vi "Configure USB Address.vi"(5 "Retry Attempts (0)":i32 min=0, 7 "Current Address (-1)":i32=-1, 8 "error in (no error)":errorcluster, 10 "New Address":i32, 11 "VISA resource name (in)":refnum<visa-resource-name>) -> (0 "error out":errorcluster, 2 "Response Cluster":T1 {"Command ID" format="%x"}, 3 "VISA resource name (out)":refnum<visa-resource-name>)   [LabVIEW 2020, in "Omega Platinum Series.lvlib"]
doc: "Change the serial address of a controller. Must be in the range 0-199 (decimal)"
uses:
  Omega Platinum Series.lvlib
  Type Defs/Response.ctl
panel:
  out "Command":string
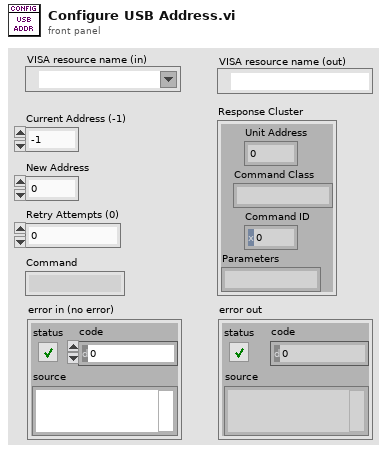
[diagram p1: front panel]
types:
  T1 = typedef "Omega Platinum Series.lvlib/Response.ctl" = cluster{"Unit Address":i32, "Command Class":string, "Command ID":u32, "Parameters":string}
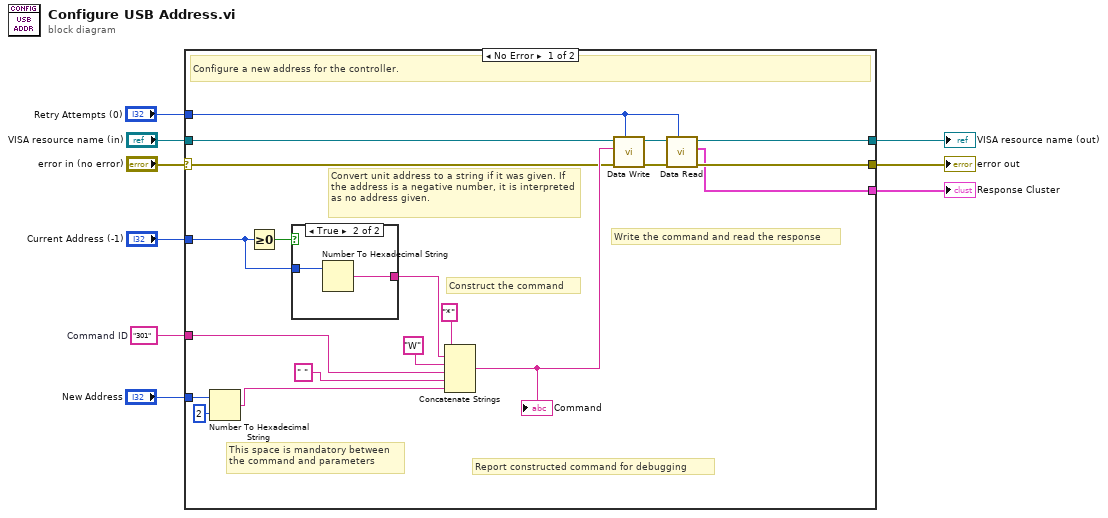
[diagram p0: block diagram]
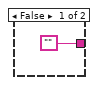
[diagram p2: hidden frame]
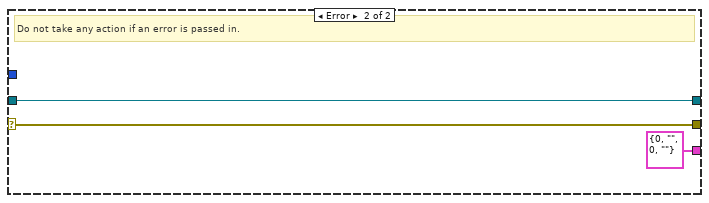
[diagram p3: hidden frame]
diagram:
  w9 = "301"  # Command ID
  n1 = case shown="No Error" "error in (no error)" {
    selector: "error in (no error)" -> [w22 w34]
    tunnel: w9 -> [w15 _]
    tunnel: "Current Address (-1)" -> [w26 _]
    tunnel: [w18 w34] -> w6
    tunnel: "VISA resource name (in)" -> [w24 w33]
    tunnel: [w19 w33] -> w4
    tunnel: [w17 T1 {"Unit Address"=0, "Command Class"="", "Command ID"=0, "Parameters"=""} ("Response Cluster")] -> w3
    tunnel: "New Address" -> [w13 _]
    tunnel: "Retry Attempts (0)" -> [w10 _]
    frame No Error {
      # "Report constructed command for debugging"
      # "Write the command and read the response"
      # "This space is mandatory between\nthe command and parameters"
      # "Convert unit address to a string if it was given. If the address is a negative number, it is interpreted as no address given."
      # "Construct the command"
      # "Configure a new address for the controller."
      n2 = Number To Hexadecimal String(1:i16 2 ("width (-)"), 2:w13) -> (0:w12:string)
      n3 = Greater Or Equal To 0?(x=w26) -> (x >= 0?=w28:bool)
      n4 = case shown="True" w28 {
        tunnel: w26 -> [_ w31]
        tunnel: ["" w30] -> w25
        frame False {
        }
        frame True {
          n5 = Number To Hexadecimal String(2:w31) -> (0:w30:string)  [unwired: 1 in]
        }
      }
      n6 = Concatenate Strings("*" ("string"), w25, "W" ("string"), w15, " " ("string"), w12) -> (w23:string)
      "Command" <- w23
      n7 = call "Data Write.vi"("Retry Attempts (0)"=w10, "error in (no error)"=w22, "Command"=w23, "VISA Refnum in"=w24) -> ("error out"=w21:errorcluster, "VISA Refnum out"=w20:refnum<visa-resource-name>)  [unwired: 6 in]
      n8 = call "Data Read.vi"("Retry Attempts (0)"=w10, "error in (no error)"=w21, "VISA Refnum in"=w20) -> ("error out"=w18:errorcluster, "Response Cluster"=w17:T1, "VISA Refnum out"=w19:refnum<visa-resource-name>)  [unwired: 5 in, 1 out]
    }
    frame Error {
      # "Do not take any action if an error is passed in."
    }
  }
  "error out" <- w6
  "VISA resource name (out)" <- w4
  "Response Cluster" <- w3
